vi "Release Queue.vi"(8 "error in (no error)":errorcluster, 11 "queue in":refnum<queue>) -> (0 "error out":errorcluster)   [LabVIEW 2018, in "ED Queued State Machine.lvlib"]
uses:
  ED Queued State Machine.lvlib
  State and Data--cluster.ctl
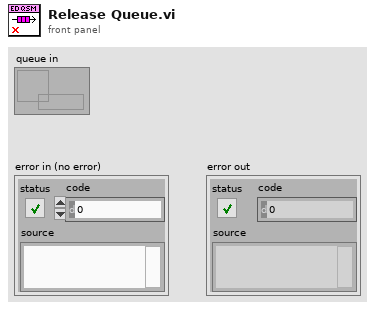
[diagram p1: front panel]
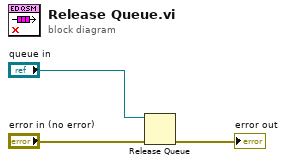
[diagram p0: block diagram]
diagram:
  n1 = Release Queue(queue="queue in", error in (no error)="error in (no error)") -> (error out=→"error out":errorcluster)  [unwired: 1 in, 2 out]
